vi "Loop (Crash Files).vi"   [LabVIEW 2019]
uses:
  Type Defs/Crash File Mode.ctl
  Type Defs/Crash File State.ctl
  Real-Time/Controls/RT FIFO Mode.ctl
  Pump 1 RT FIFO.vi
  Pump 2 RT FIFO.vi
  Pump 3 RT FIFO.vi
  Pump 4 RT FIFO.vi
  Pump 5 RT FIFO.vi
  Pump 6 RT FIFO.vi
types:
  T1 = typedef "Crash File Mode.ctl" = enum16{"Pump 1 Write", "Pump 2 Write", "Pump 3 Write", "Pump 4 Write", "Pump 5 Write", "Pump 6 Write", "Read All", "Init"}
  T2 = typedef "Crash File State.ctl" = enum16{"Idle", "Alarm Triggered", "Alarm Latched"}
  T3 = typedef "RT FIFO Mode.ctl" = enum16{"Create", "Write", "Read", "Delete"}
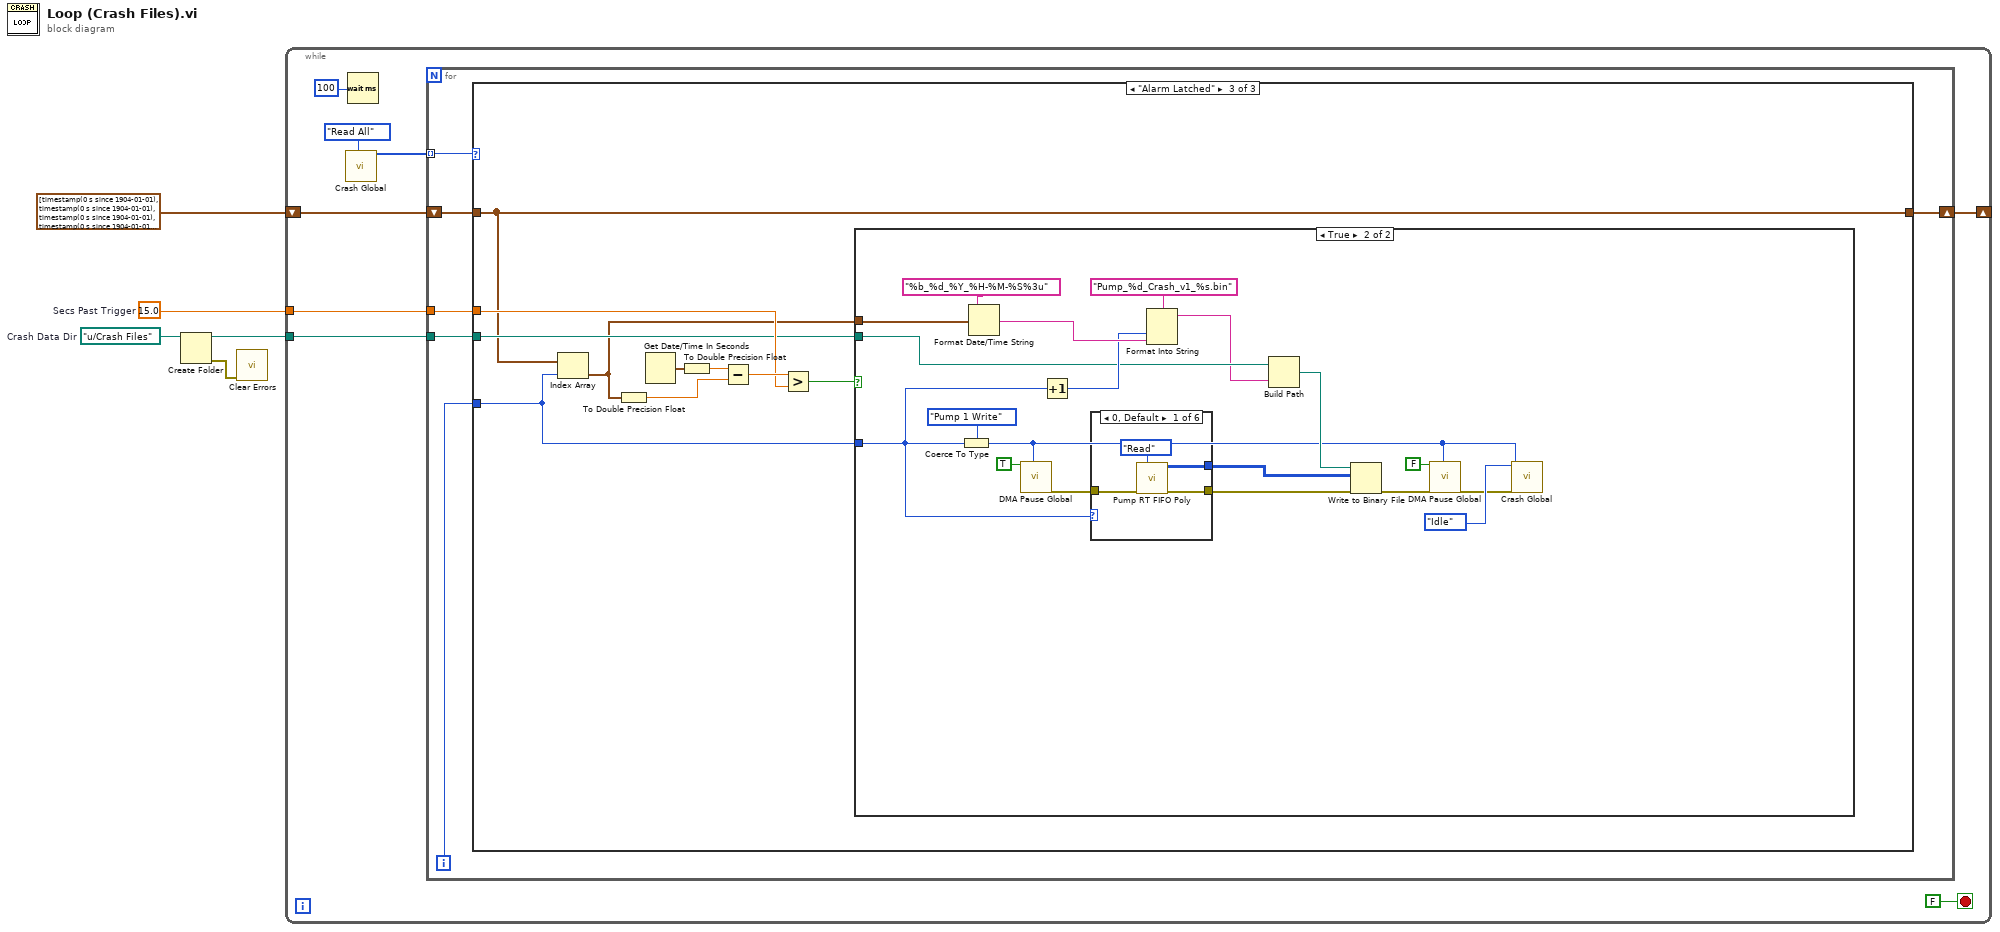
[diagram p0: block diagram]
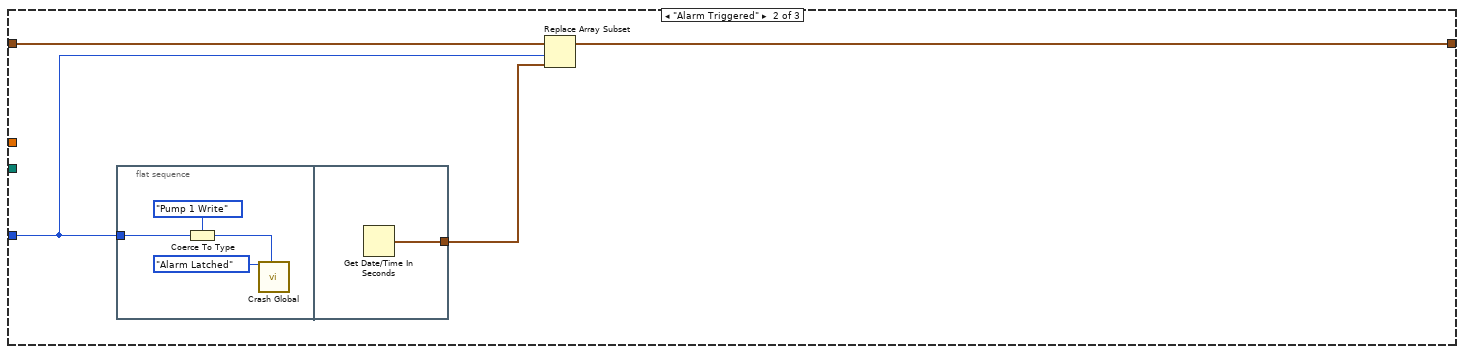
[diagram p3: hidden frame]
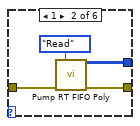
[diagram p5: hidden frame]
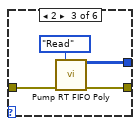
[diagram p6: hidden frame]
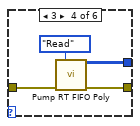
[diagram p7: hidden frame]
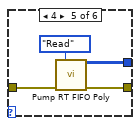
[diagram p8: hidden frame]
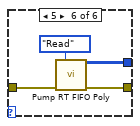
[diagram p9: hidden frame]
diagram:
  w3 = path "u:/Crash Files"  # Crash Data Dir
  w4 = 15.0  # Secs Past Trigger
  n1 = Create Folder(path (use dialog)=w3) -> (created path=w2:path, error out=w1:errorcluster)  [unwired: 2 in, 1 out]
  n2 = call <vilib>:"Clear Errors.vi"("error in (no error)"=w1) -> ()  [unwired: 5 in, 2 out]
  n3 = while {
    shift-right: [w9] -> _
    shift-left: timestamp[] [timestamp(0 s since 1904-01-01), timestamp(0 s since 1904-01-01), timestamp(0 s since 1904-01-01), timestamp(0 s since 1904-01-01), timestamp(0 s since 1904-01-01), timestamp(-21600 s since 1904-01-01)] -> [w8]
    tunnel: w4 -> [w7]
    tunnel: w2 -> [w6]
    stop <- FALSE stop-if-true
    n4 = call "Crash Global.vi"("Mode"=Crash_File_Mode."Read All") -> ("Crash File States"=w10:T2[])  [unwired: 17 in, 1 out]
    n5 = Wait (ms)(milliseconds to wait=u32 100) -> ()  [unwired: 1 out]
    n6 = for {
      tunnel: w10 -> [w19] mode=indexing
      shift-right: [w17] -> w9
      shift-left: w8 -> [w16]
      tunnel: w7 -> [w15]
      tunnel: w6 -> [w14]
      i -> [w18]
      n7 = case shown="\"Alarm Latched\"" w19 {
        tunnel: w18 -> [_ w23 w35]
        tunnel: [w20 w21 w32] -> w17
        tunnel: w16 -> [w20 w24 w32]
        tunnel: w15 -> [_ _ w34]
        tunnel: w14 -> [_ _ w33]
        frame "Idle", Default {
        }
        frame "Alarm Triggered" {
          n8 = flat-sequence {
            tunnel: w23 -> [w28]
            tunnel: [w29] -> w22
            frame #0 {
              n9 = Coerce To Type(0:w28, 1:Crash_File_Mode."Pump 1 Write" ("Mode")) -> (2:w25:T1)
              n10 = call "Crash Global.vi"("Crash State IN"=Crash_File_State."Alarm Latched", "Mode"=w25) -> ()  [unwired: 16 in, 2 out]
            }
            frame #1 {
              n11 = Get Date/Time In Seconds() -> (seconds since 1Jan1904=w29:timestamp)
            }
          }
          n12 = Replace Array Subset(array=w24, new element=w22, index=w23) -> (w21:timestamp[])
        }
        frame "Alarm Latched" {
          n13 = Index Array(array=w32, index=w35) -> (element=w30:timestamp)
          n14 = To Double Precision Float(number=w30) -> (double precision float=w31:dbl)
          n15 = Get Date/Time In Seconds() -> (seconds since 1Jan1904=w39:timestamp)
          n16 = To Double Precision Float(number=w39) -> (double precision float=w38:dbl)
          n17 = Subtract(x=w38, y=w31) -> (x-y=w37:dbl)
          n18 = Greater?(x=w37, y=w34) -> (0:w36:bool)
          n19 = case shown="True" w36 {
            tunnel: w35 -> [_ w49]
            tunnel: w33 -> [_ w47]
            tunnel: w30 -> [_ w53]
            frame False {
            }
            frame True {
              n20 = Coerce To Type(0:w49, 1:Crash_File_Mode."Pump 1 Write" ("Mode")) -> (2:w42:T1)
              n21 = Format Date/Time String(time format string (%c)="%b_%d_%Y_%H-%M-%S%3u", seconds (now)=w53) -> (date/time string=w50:string)  [unwired: 1 in]
              n22 = call "DMA Pause Global.vi"("Pause IN"=TRUE, "Mode"=w42) -> ("Error OUT"=w56:errorcluster)  [unwired: 16 in, 1 out]
              n23 = Increment(x=w49) -> (x+1=w48:i32)
              n24 = case shown="0, Default" w49 {
                tunnel: w56 -> [w61 w65 w69 w73 w77 w81]
                tunnel: [w59 w63 w67 w71 w75 w80] -> w54
                tunnel: [w60 w64 w68 w72 w76 w79] -> w55
                frame 0, Default {
                  n25 = call-poly "Pump RT FIFO Poly.vi"("Mode (Write)"=RT_FIFO_Mode."Read" ("Mode"), "Error IN"=w61) -> ("Data OUT"=w60:u16[][], "Error OUT"=w59:errorcluster)  [unwired: 12 in]
                }
                frame 1 {
                  n26 = call-poly "Pump RT FIFO Poly.vi"("Mode (Write)"=RT_FIFO_Mode."Read" ("Mode"), "Error IN"=w65) -> ("Data OUT"=w64:u16[][], "Error OUT"=w63:errorcluster)  [unwired: 12 in]
                }
                frame 2 {
                  n27 = call-poly "Pump RT FIFO Poly.vi"("Mode (Write)"=RT_FIFO_Mode."Read" ("Mode"), "Error IN"=w69) -> ("Data OUT"=w68:u16[][], "Error OUT"=w67:errorcluster)  [unwired: 12 in]
                }
                frame 3 {
                  n28 = call-poly "Pump RT FIFO Poly.vi"("Mode (Write)"=RT_FIFO_Mode."Read" ("Mode"), "Error IN"=w73) -> ("Data OUT"=w72:u16[][], "Error OUT"=w71:errorcluster)  [unwired: 12 in]
                }
                frame 4 {
                  n29 = call-poly "Pump RT FIFO Poly.vi"("Mode (Write)"=RT_FIFO_Mode."Read" ("Mode"), "Error IN"=w77) -> ("Data OUT"=w76:u16[][], "Error OUT"=w75:errorcluster)  [unwired: 12 in]
                }
                frame 5 {
                  n30 = call-poly "Pump RT FIFO Poly.vi"("Mode (Write)"=RT_FIFO_Mode."Read" ("Mode"), "Error IN"=w81) -> ("Data OUT"=w79:u16[][], "Error OUT"=w80:errorcluster)  [unwired: 12 in]
                }
              }
              n31 = Format Into String(format string="Pump_%d_Crash_v1_%s.bin", w48, w50) -> (resulting string=w46:string)  [unwired: 2 in, 1 out]
              n32 = Build Path(base path=w47, name or relative path=w46) -> (appended path=w45:path)
              n33 = Write to Binary File(file (use dialog)=w45, data=w55, error in=w54) -> (error out=w43:errorcluster)  [unwired: 3 in, 2 out]
              n34 = call "DMA Pause Global.vi"("Pause IN"=FALSE, "Error IN"=w43, "Mode"=w42) -> ("Error OUT"=w40:errorcluster)  [unwired: 15 in, 1 out]
              n35 = call "Crash Global.vi"("Crash State IN"=Crash_File_State."Idle", "Error IN"=w40, "Mode"=w42) -> ()  [unwired: 15 in, 2 out]
            }
          }
        }
      }
    }
  }
